vi "Write Store.vi"(8 "error in (no error)":errorcluster, 10 "Store":T1, 11 "AReceipt in":refnum<class "AReceipt.lvclass">) -> (0 "error out":errorcluster, 3 "AReceipt out":refnum<class "AReceipt.lvclass">)   [LabVIEW 2020, in "AReceipt.lvclass"]
uses:
  AReceipt.lvclass
  AReceipt.lvclass/AReceipt.ctl
  Store STYP.ctl
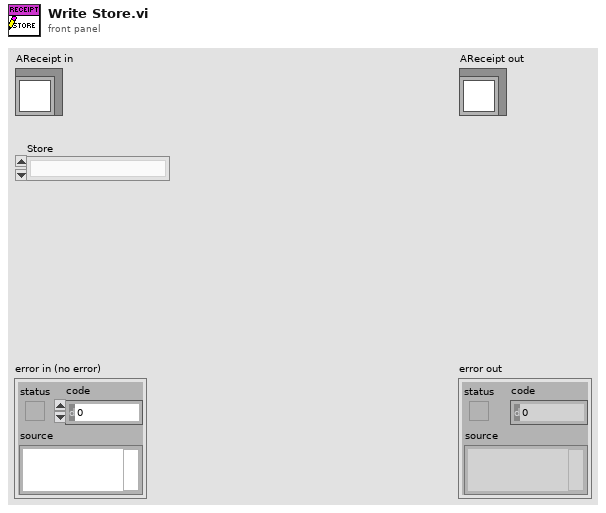
[diagram p1: front panel]
types:
  T1 = typedef "AReceipt.lvclass/Store STYP.ctl" = enum16{""}
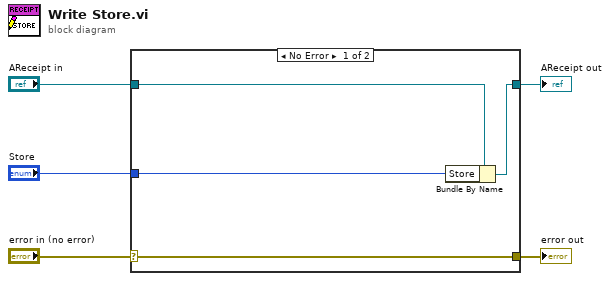
[diagram p0: block diagram]
diagram:
  n1 = case shown="No Error" "error in (no error)" {
    selector: "error in (no error)" -> [w9 w10]
    tunnel: [w9 w10] -> w4
    tunnel: [w7 w11] -> w2
    tunnel: "AReceipt in" -> [w8 w11]
    tunnel: "Store" -> [w6 _]
    frame No Error {
      n2 = Bundle By Name(cluster=w8, "Store"=w6) -> (w7:refnum<class "AReceipt.lvclass">)
    }
    frame Error {
    }
  }
  "error out" <- w4
  "AReceipt out" <- w2
